vi "JustReadCurrent.vi"(8 "error in (no error)":errorcluster, 10 "Function (0: Volts)":u16=1, 11 "Keithley In":refnum<visa-resource-name>) -> (0 "error out":errorcluster, 2 "Measured Current":dbl, 3 "Keithley Out":refnum<visa-resource-name>)   [LabVIEW 2013]
uses:
  <instrlib>/Keithley 24XX/Public/Data/Read (Single Point).vi
  <instrlib>/Keithley 24XX/Keithley 24XX.lvlib
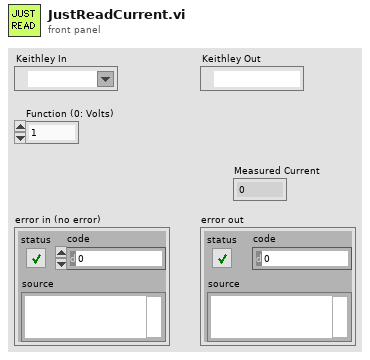
[diagram p1: front panel]
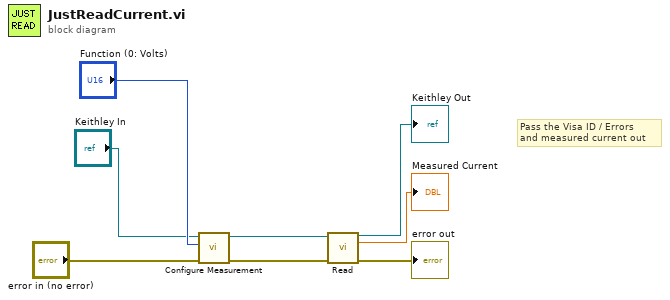
[diagram p0: block diagram]
diagram:
  # "Pass the Visa ID / Errors \nand measured current out"
  n1 = call <instrlib>:"Configure Measurement.vi"("error in (no error)"="error in (no error)", "Function (0: Volts)"="Function (0: Volts)", "VISA resource name"="Keithley In") -> ("error out"=w1:errorcluster, "VISA resource name out"=w2:refnum<visa-resource-name>)  [unwired: 7 in]
  n2 = call-poly <instrlib>:"Read.vi"("VISA resource name"=w2, "error in (no error)"=w1) -> ("VISA resource name out"=→"Keithley Out":refnum<visa-resource-name>, "Current"=→"Measured Current":sgl, "error out"=→"error out":errorcluster)  [unwired: 7 in, 4 out]
